vi "PostCopyScripting.vi"(10 "MetaDataObj":refnum<class "MetaDataObj.lvclass">, 11 "User Project":refnum<vi>) -> ()   [LabVIEW 2014, in "SequencerActionScript.lvclass"]
doc: "NI Tag Bus Module Framework 1.0.2.36\nNI Systems Engineering"
uses:
  SequencerActionScript.lvclass
  <resource>/dialog/NewProjectWizard/MetaDataObj/MetaDataObj.lvclass
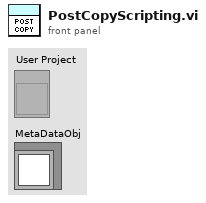
[diagram p1: front panel]
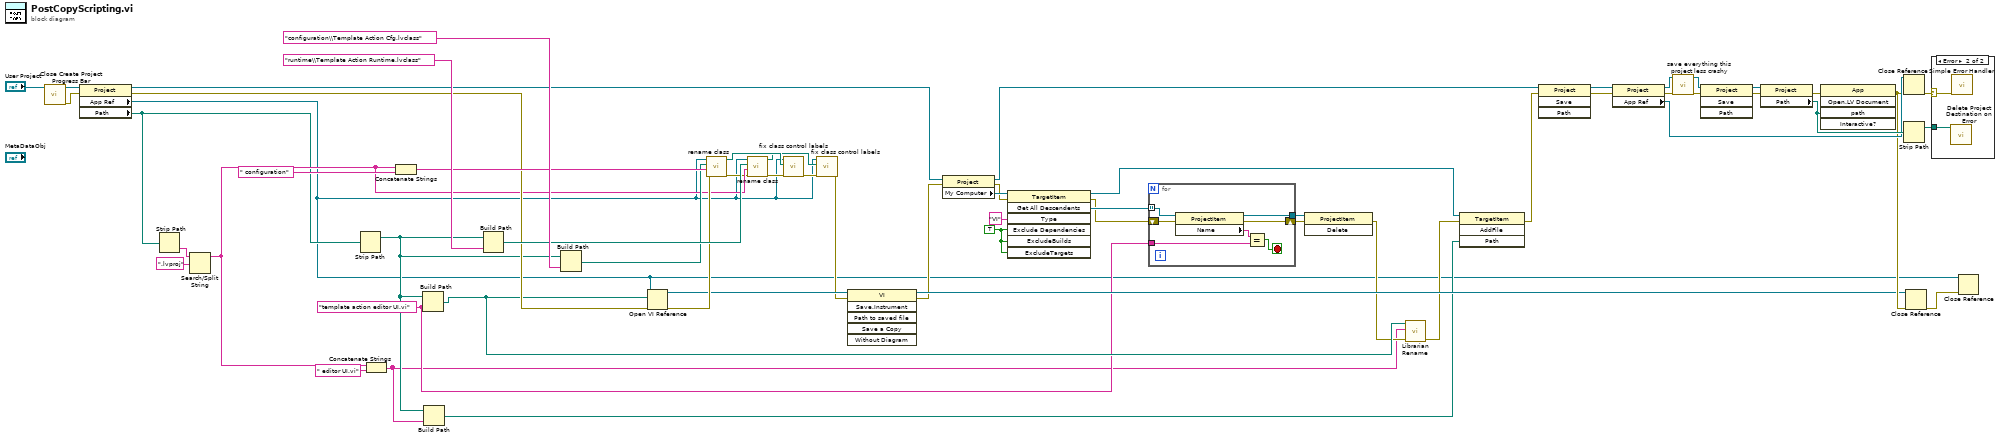
[diagram p0: block diagram]
diagram:
  w23 = TRUE ("ExcludeDependencies")
  w21 = "template action editor UI.vi" ("name or relative path")
  n1 = call <resource>:"Close Create Project Progress Bar.vi"("Project"="User Project") -> ("error out"=w1:errorcluster, "dup Project"=w2:refnum<vi>)  [unwired: 9 in]
  n2 = property class="Project"(reference=w2, error in=w1) -> (reference out=w26:refnum<vi>, error out=w38:errorcluster, "App Ref"=w4:refnum<vi>, "Path"=w5:path)
  n3 = Strip Path(path=w5) -> (name=w31:string)  [unwired: 1 out]
  n4 = Search/Split String(string=w31, search string/char (-)=".lvproj") -> (substring before match=w30:string)  [unwired: 1 in, 2 out]
  n5 = Strip Path(path=w5) -> (stripped path=w13:path)  [unwired: 1 out]
  n6 = Concatenate Strings(w30, " editor UI.vi" ("string")) -> (w12:string)
  n7 = Concatenate Strings(w30, " configuration" ("string")) -> (w43:string)
  n8 = Build Path(base path=w13, name or relative path=w21) -> (appended path=w28:path)
  n9 = Build Path(base path=w13, name or relative path=w12) -> (appended path=w11:path)
  n10 = Build Path(base path=w13, name or relative path="runtime\\Template Action Runtime.lvclass") -> (appended path=w45:path)
  n11 = Build Path(base path=w13, name or relative path="configuration\\Template Action Cfg.lvclass") -> (appended path=w42:path)
  n12 = Open VI Reference(application reference (local)=w4, vi path=w28, error in (no error)=w38) -> (vi reference=w33:refnum<vi>, error out=w37:errorcluster)  [unwired: 3 in]
  n13 = call "rename class.vi"("error in"=w37, "new name"=w43, "class path"=w42, "application in"=w4) -> ("error out"=w7:errorcluster, "new library path"=w41:path)  [unwired: 6 in]
  n14 = call "rename class.vi"("error in"=w7, "new name"=w30, "class path"=w45, "application in"=w4) -> ("error out"=w6:errorcluster, "new library path"=w39:path)  [unwired: 6 in]
  n15 = call "fix class control labels.vi"("error in"=w6, "class to load"=w41, "application in"=w4) -> ("error out"=w40:errorcluster)  [unwired: 8 in]
  n16 = call "fix class control labels.vi"("error in"=w40, "class to load"=w39, "application in"=w4) -> ("error out"=w29:errorcluster)  [unwired: 8 in]
  n17 = invoke class="VI" method="Save.Instrument"(reference=w33, error in=w29) -> (reference out=w35:refnum<vi>, error out=w19:errorcluster)  [unwired: 4 in, 4 out]
  n18 = property class="Project"(reference=w26, error in=w19) -> (reference out=w25:refnum<vi>, error out=w18:errorcluster, "My Computer"=w27:refnum<vi>)
  n19 = invoke class="TargetItem" method="Get All Descendents"(reference=w27, error in=w18, "Type"="VI", "Exclude Dependencies"=w23, "ExcludeBuilds"=w23, "ExcludeTargets"=w23) -> (reference out=w10:refnum<vi>, error out=w17:errorcluster, "All Descendents"=w22:refnum<vi>[])  [unwired: 1 in, 4 out]
  n20 = for {
    tunnel: w22 -> [w67] mode=indexing
    tunnel: w21 -> [w65]
    tunnel: [w63] -> w20
    shift-right: [w61] -> w16
    shift-left: w17 -> [w62]
    stop <- w64 stop-if-true
    n21 = property class="ProjectItem"(reference=w67, error in=w62) -> (reference out=w63:refnum<vi>, error out=w61:errorcluster, "Name"=w66:string)
    n22 = Equal?(x=w66, y=w65) -> (x = y?=w64:bool)
  }
  n23 = invoke class="ProjectItem" method="Delete"(reference=w20, error in=w16) -> (error out=w15:errorcluster)  [unwired: 1 in, 2 out]
  n24 = call <vilib>:"Librarian Rename.vi"("error in (no error)"=w15, "new name"=w12, "path"=w28) -> ("error out"=w14:errorcluster)  [unwired: 7 in, 1 out]
  n25 = invoke class="TargetItem" method="AddFile"(reference=w10, error in=w14, "Path"=w11) -> (error out=w9:errorcluster)  [unwired: 1 in, 3 out]
  n26 = invoke class="Project" method="Save"(reference=w25, error in=w9) -> (reference out=w54:refnum<vi>, error out=w53:errorcluster)  [unwired: 2 in, 2 out]
  n27 = property class="Project"(reference=w54, error in=w53) -> (reference out=w51:refnum<vi>, error out=w52:errorcluster, "App Ref"=w50:refnum<vi>)
  n28 = call "save everything this project less crashy.vi"("error in"=w52, "project in"=w51) -> ("error out"=w56:errorcluster, "project out"=w55:refnum<vi>)  [unwired: 8 in]
  n29 = invoke class="Project" method="Save"(reference=w55, error in=w56) -> (reference out=w58:refnum<vi>, error out=w59:errorcluster)  [unwired: 2 in, 2 out]
  n30 = property class="Project"(reference=w58, error in=w59) -> (error out=w60:errorcluster, "Path"=w57:path)  [unwired: 1 out]
  n31 = invoke class="App" method="Open.LV Document"(error in=w60, "path"=w57) -> (error out=w36:errorcluster)  [unwired: 3 in, 4 out]
  n32 = Close Reference(reference=w50, error in (no error)=w36) -> (error out=w49:errorcluster)
  n33 = Strip Path(path=w57) -> (stripped path=w48:path)  [unwired: 1 out]
  n34 = Close Reference(reference=w35, error in (no error)=w36) -> (error out=w8:errorcluster)
  n35 = case shown="Error" w49 {
    selector: w49 -> [_ w68]
    tunnel: w48 -> [_ w69]
    frame No Error {
    }
    frame Error {
      n36 = call <resource>:"Delete Project Destination on Error.vi"("Project Destination Root"=w69) -> ()  [unwired: 11 in]
      n37 = call <vilib>:"Simple Error Handler.vi"("error in (no error)"=w68) -> ()  [unwired: 4 in, 5 out]
    }
  }
  n38 = Close Reference(reference=w4, error in (no error)=w8) -> ()  [unwired: 1 out]
